vi "Redraw All Icons.vi"(8 "error in (no error)":errorcluster, 11 "Toolbar Control in":refnum<class "Toolbar Control.lvclass">) -> (0 "error out":errorcluster, 2 "Toolbar Image":picture, 3 "Toolbar Control out":refnum<class "Toolbar Control.lvclass">)   [LabVIEW 2011, in "Toolbar Control.lvclass"]
doc: "This VI will cause all icons to be redrawn, and to display them on <B>Toolbar Image</B>.\n\n-------------\nDeveloped by Brian Hoover (hooovahh)"
uses:
  Toolbar Control.lvclass
  Toolbar Control.lvclass/Toolbar Control.ctl
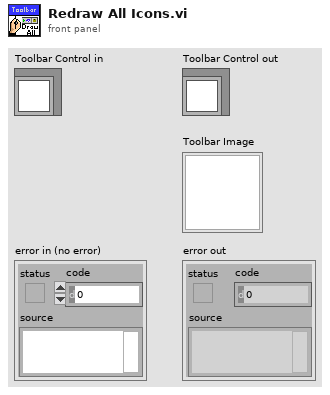
[diagram p1: front panel]
types:
  T1 = typedef "Toolbar Control.lvclass/Icon Data.ctl" = cluster{"Original Image Path":path, "Original Image Data":T2, "Scaled Icon":picture, "Button Name":string, "Button State":T3, "Icon Type":T4}
  T2 = typedef "imagedata.ctl" = cluster{"image type":i32, "image depth":i32, "image":u8[], "mask":u8[], "colors":u32[], "Rectangle":cluster{"left":i16, "top":i16, "right":i16, "bottom":i16}}
  T3 = typedef "Toolbar Control.lvclass/Button State.ctl" = enum8{"Enabled", "Disabled", "Disabled and Grayed Out"}
  T4 = typedef "Icon Type.ctl" = enum16{"Normal Icon", "Separator Icon", "More Options"}
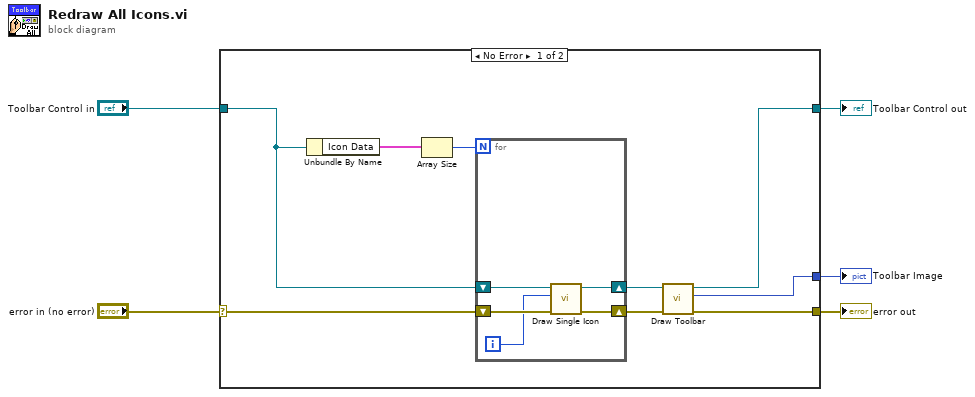
[diagram p0: block diagram]
diagram:
  n1 = case shown="No Error" "error in (no error)" {
    selector: "error in (no error)" -> [w14 w21]
    tunnel: [w8 w21] -> w4
    tunnel: [w7 w20] -> w2
    tunnel: "Toolbar Control in" -> [w11 w20]
    tunnel: [w6 _] -> w1
    frame No Error {
      n2 = Unbundle By Name(w11) -> ("Icon Data"=w13:T1[])
      n3 = Array Size(array=w13) -> (size(s)=w12:i32)
      n4 = for {
        N: w12 -> [_]
        shift-right: [w18] -> w10
        shift-left: w11 -> [w19]
        shift-right: [w16] -> w9
        shift-left: w14 -> [w17]
        i -> [w15]
        n5 = call "Draw Single Icon.vi"("error in (no error)"=w17, "Icon Index"=w15, "Toolbar Control in"=w19) -> ("error out"=w16:errorcluster, "Toolbar Control out"=w18:refnum<class "Toolbar Control.lvclass">)  [unwired: 7 in]
      }
      n6 = call "Draw Toolbar.vi"("error in (no error)"=w9, "Toolbar Control in"=w10) -> ("error out"=w8:errorcluster, "Toolbar Image"=w6:picture, "Toolbar Control out"=w7:refnum<class "Toolbar Control.lvclass">)  [unwired: 7 in]
    }
    frame Error {
    }
  }
  "error out" <- w4
  "Toolbar Control out" <- w2
  "Toolbar Image" <- w1
